vi "length of a given number.vi"(11 "Numeric in":dbl) -> (3 "Numeric out":i32)   [LabVIEW 2020]
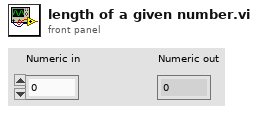
[diagram p1: front panel]
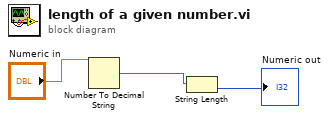
[diagram p0: block diagram]
diagram:
  n1 = Number To Decimal String(number="Numeric in") -> (decimal integer string=w1:string)  [unwired: 1 in]
  n2 = String Length(string=w1) -> (length=→"Numeric out":i32)
